vi "Set controls.vi"(8 "error in (no error)":errorcluster, 10 "Parameters":T1={"Start frequency"=500000.0, "End frequency"=2000000.0, "Number of points"=38000, "Amplitude"=2.1, "Work folder"=path "C:/Data/RUS"} {"Amplitude" format="%#_6p"; "End frequency" format="%#_6p"; "Start frequency" format="%#_6p"}, 11 "RUS Measurement in":refnum<class "RUS Measurement.lvclass">) -> (0 "error out":errorcluster, 3 "RUS Measurement out":refnum<class "RUS Measurement.lvclass">)   [LabVIEW 2014, in "RUS Measurement.lvclass"]
uses:
  RUS Measurement.lvclass
  RUS Parameters.ctl
  RUS/Controls/Sweep settings.ctl
  RUS Measurement.lvclass/RUS Measurement.ctl
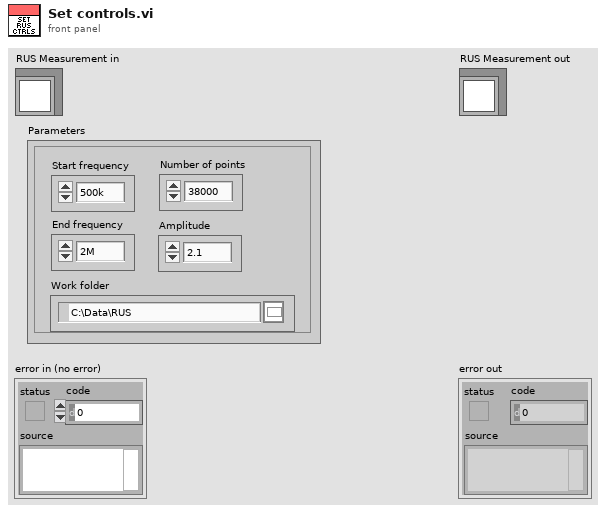
[diagram p1: front panel]
types:
  T1 = typedef "RUS Parameters.ctl" = cluster{"Start frequency":dbl, "End frequency":dbl, "Number of points":i32, "Amplitude":dbl, "Work folder":path}
  T2 = typedef "Sweep settings.ctl" = cluster{"Update rate (Hz)":dbl, "Start F, Hz":dbl, "Stop F":dbl, "Number of points":i32, "Amplitude":dbl, "Init&amplitude":bool, "IF":dbl, "Time constant":dbl}
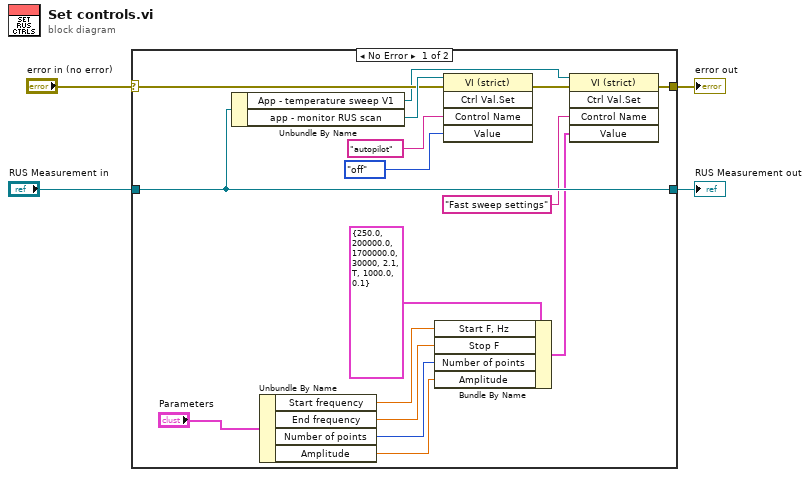
[diagram p0: block diagram]
diagram:
  n1 = case shown="No Error" "error in (no error)" {
    selector: "error in (no error)" -> [w16 w22]
    tunnel: [w8 w22] -> w3
    tunnel: [w20 w21] -> w1
    tunnel: "RUS Measurement in" -> [w20 w21]
    frame No Error {
      n2 = Unbundle By Name(w20) -> ("App - temperature sweep V1"=w15:refnum<vi>, "app - monitor RUS scan"=w19:refnum<vi>)
      n3 = Unbundle By Name("Parameters") -> ("Start frequency"=w12:dbl, "End frequency"=w7:dbl, "Number of points"=w6:i32, "Amplitude"=w5:dbl)
      n4 = Bundle By Name(cluster=T2 {"Update rate (Hz)"=250.0, "Start F, Hz"=200000.0, "Stop F"=1700000.0, "Number of points"=30000, "Amplitude"=2.1, "Init&amplitude"=TRUE, "IF"=1000.0, "Time constant"=0.1} ("Fast swep settings"), "Start F, Hz"=w12, "Stop F"=w7, "Number of points"=w6, "Amplitude"=w5) -> (w11:T2)
      n5 = invoke class="VI (strict)" method="Ctrl Val.Set"(reference=w19, error in=w16, "Control Name"="autopilot", "Value"=enum32{"on", "off"}."off" ("autopilot")) -> (error out=w9:errorcluster)  [unwired: 1 in, 4 out]
      n6 = invoke class="VI (strict)" method="Ctrl Val.Set"(reference=w15, error in=w9, "Control Name"="Fast sweep settings", "Value"=w11) -> (error out=w8:errorcluster)  [unwired: 1 in, 4 out]
    }
    frame Error {
    }
  }
  "error out" <- w3
  "RUS Measurement out" <- w1
